vi "Check Subscription Policy.vi"(8 "error in (no error)":errorcluster, 11 "Subscription Policy Reference":T1) -> (0 "error out (Unsubscribe?)":errorcluster)   [LabVIEW 2015, in "IMediator.lvlib" / "ISubscriptionPolicy.lvclass"]
doc: "This method decides whether or not to send or otherwise handle the new data value. The policy is set and maintained by the subscriber. The Topic Actor knows no policy details, it just passes the new value in. If there is a failure inside this method, the Topic Actor must assume the listener is no longer valid (dead/unrecoverable) and should delete it from the Subscriber list.\n\n<License>\nCopyright © 2017 Composed Systems, LLC | All rights reserved\nwww.composed.io\n\nAuthor: Ethan Stern <ethan.stern@composed.io>\n\nThis software is provided \"AS IS\" WITHOUT WARRANTIES, either express or implied, AND IS FOR EDUCATIONAL PURPOSES ONLY.\n</License>"
uses:
  ISubscriptionPolicy.lvclass
  ISubscriptionPolicy Reference.ctl
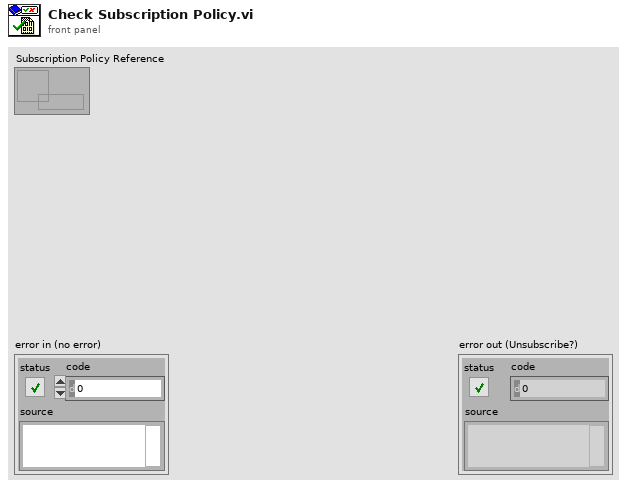
[diagram p1: front panel]
types:
  T1 = typedef "IMediator.lvlib/ISubscriptionPolicy.lvclass/ISubscriptionPolicy Reference.ctl" = refnum<data-value>
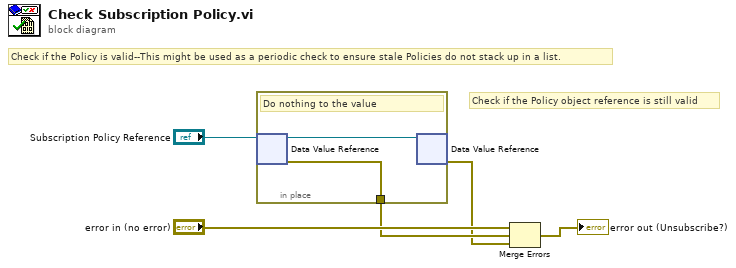
[diagram p0: block diagram]
diagram:
  # "Check if the Policy object reference is still valid"
  # "Check if the Policy is valid--This might be used as a periodic check to ensure stale Policies do not stack up in a list."
  n1 = in-place {
    in-place-border: [w6] -> w2
    # "Do nothing to the value"
    n2 = in-place-dvr #1("Subscription Policy Reference") -> (w7:refnum<class "ISubscriptionPolicy.lvclass">, w6:errorcluster)
    n3 = in-place-dvr #1(w7) -> (w1:errorcluster)  [unwired: 1 out]
  }
  n4 = Merge Errors("error in (no error)", w2, w1) -> (→"error out (Unsubscribe?)":errorcluster)
